vi "connectTask.vi"(8 "error in (no error)":errorcluster, 10 "pathLvLib":path, 11 "pathMonitor":path) -> (0 "error out":errorcluster)   [LabVIEW 2018]
doc: "Task of the connection of LabVIEW."
uses:
  SalProcess/SalProcess.lvclass
  LibReader/LibReader.lvclass
  SalProcess/SalProcess.lvclass/SalProcess.ctl
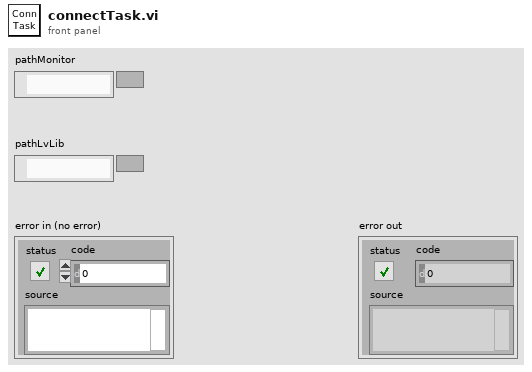
[diagram p1: front panel]
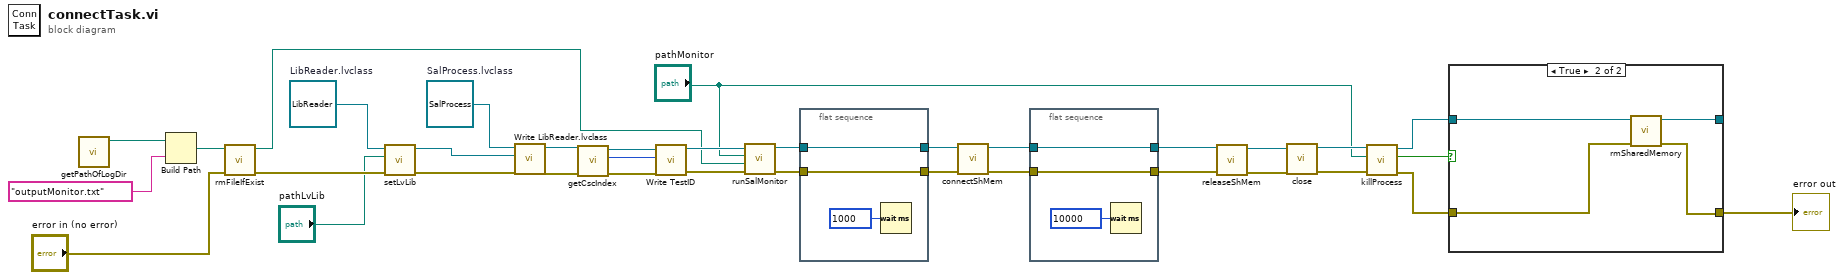
[diagram p0: block diagram]
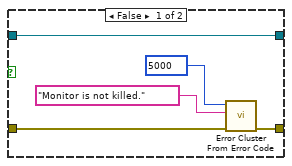
[diagram p2: hidden frame]
diagram:
  w22 = refnum<class "LibReader.lvclass"> refnum  # LibReader.lvclass
  w21 = refnum<class "SalProcess.lvclass"> refnum  # SalProcess.lvclass
  n1 = call "getPathOfLogDir.vi"() -> ("logDirPath"=w35:path)  [unwired: 11 in]
  n2 = Build Path(base path=w35, name or relative path="outputMonitor.txt") -> (appended path=w33:path)
  n3 = call "rmFileIfExist.vi"("error in (no error)"="error in (no error)", "path"=w33) -> ("error out"=w20:errorcluster, "pathDup"=w29:path)  [unwired: 8 in]
  n4 = call "setLvLib.vi"("error in (no error)"=w20, "pathLvLib"="pathLvLib", "LibReader in"=w22) -> ("error out"=w19:errorcluster, "LibReader out"=w18:refnum<class "LibReader.lvclass">)  [unwired: 7 in]
  n5 = call "Write LibReader.lvclass.vi"("error in (no error)"=w19, "LibReader.lvclass"=w18, "SalProcess in"=w21) -> ("error out"=w1:errorcluster, "SalProcess out"=w5:refnum<class "SalProcess.lvclass">)  [unwired: 7 in]
  n6 = call "getCscIndex.vi"("error in (no error)"=w1, "SalProcess in"=w5) -> ("error out"=w2:errorcluster, "cscIdx"=w3:i32, "SalProcess out"=w4:refnum<class "SalProcess.lvclass">)  [unwired: 7 in]
  n7 = call "Write TestID.vi"("error in (no error)"=w2, "TestID"=w3, "SalProcess in"=w4) -> ("error out"=w30:errorcluster, "SalProcess out"=w31:refnum<class "SalProcess.lvclass">)  [unwired: 7 in]
  n8 = call "runSalMonitor.vi"("error in (no error)"=w30, "pathOfOutput"=w29, "pathOfSalMonitor"="pathMonitor", "SalProcess in"=w31) -> ("error out"=w28:errorcluster, "SalProcess out"=w27:refnum<class "SalProcess.lvclass">)  [unwired: 6 in]
  n9 = flat-sequence {
    tunnel: w28 -> [w38]
    tunnel: w27 -> [w36]
    tunnel: [w38] -> w12
    tunnel: [w36] -> w13
    frame #0 {
      n10 = Wait (ms)(milliseconds to wait=u32 1000) -> ()  [unwired: 1 out]
    }
  }
  n11 = call "connectShMem.vi"("error in (no error)"=w12, "SalProcess in"=w13) -> ("error out"=w11:errorcluster, "SalProcess out"=w10:refnum<class "SalProcess.lvclass">)  [unwired: 7 in, 1 out]
  n12 = flat-sequence {
    tunnel: w11 -> [w40]
    tunnel: w10 -> [w41]
    tunnel: [w41] -> w7
    tunnel: [w40] -> w6
    frame #0 {
      n13 = Wait (ms)(milliseconds to wait=u32 10000) -> ()  [unwired: 1 out]
    }
  }
  n14 = call "releaseShMem.vi"("error in (no error)"=w6, "SalProcess in"=w7) -> ("error out"=w8:errorcluster, "SalProcess out"=w9:refnum<class "SalProcess.lvclass">)  [unwired: 7 in, 1 out]
  n15 = call "close.vi"("error in (no error)"=w8, "SalProcess in"=w9) -> ("error out"=w16:errorcluster, "SalProcess out"=w17:refnum<class "SalProcess.lvclass">)  [unwired: 8 in]
  n16 = call "killProcess.vi"("error in (no error)"=w16, "pathOfProcess"="pathMonitor", "SalProcess in"=w17) -> ("error out"=w24:errorcluster, "isRemoved"=w26:bool, "SalProcess out"=w25:refnum<class "SalProcess.lvclass">)  [unwired: 6 in]
  n17 = case shown="True" w26 {
    tunnel: w25 -> [w46 w47]
    tunnel: w24 -> [w44 w48]
    tunnel: [w45 w50] -> w23
    tunnel: [w46 w49] -> _
    frame False {
      n18 = call <vilib>:"Error Cluster From Error Code.vi"("error in (no error)"=w44, "error message (\"\")"="Monitor is not killed." ("error message (\"\")"), "error code (0)"=5000) -> ("error out"=w45:errorcluster)  [unwired: 6 in]
    }
    frame True {
      n19 = call "rmSharedMemory.vi"("error in (no error)"=w48, "SalProcess in"=w47) -> ("error out"=w50:errorcluster, "SalProcess out"=w49:refnum<class "SalProcess.lvclass">)  [unwired: 7 in, 1 out]
    }
  }
  "error out" <- w23
